vi "Write-OSP-J-t.vi"(8 "Init cluster":T1, 11 "Array":dbl[][](array[numeric])) -> ()   [LabVIEW 2020]
uses:
  <vilib>/Utility/file.llb/Write Delimited Spreadsheet (DBL).vi
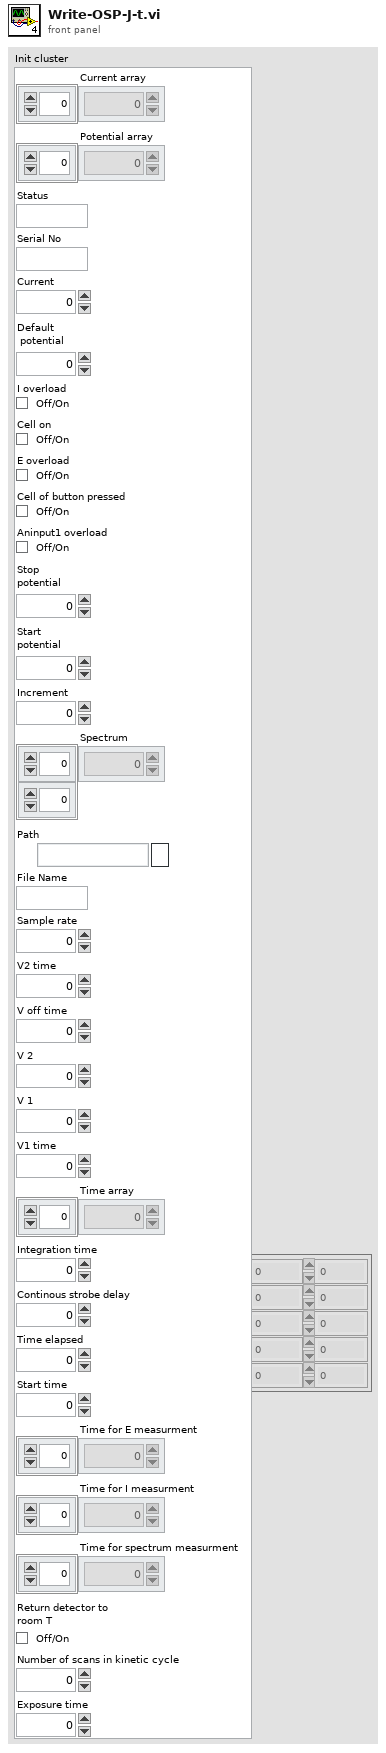
[diagram p1: front panel]
types:
  T1 = cluster{"Current array":dbl[], "Potential array":dbl[], "Status":string, "Serial No":string, "Current":dbl, "Default\n potential":dbl, "I overload":bool, "Cell on":bool, "E overload":bool, "Cell of button pressed":bool, "Aninput1 overload":bool, "Stop \npotential":dbl, "Start \npotential":dbl, "Increment":dbl, "Spectrum":dbl[][], "Path":path, "File Name":string, "Sample rate":dbl, "V2 time":dbl, "V off time":dbl, "V 2":dbl, "V 1":dbl, "V1 time":dbl, "Time array":dbl[], "Integration time":i32, "Continous strobe delay":i32, "Time elapsed ":i32, "Start time":i32, "Time for E measurment":i32[], "Time for I measurment ":i32[], "Time for spectrum measurment":i32[], "Return detector to \nroom T":bool, "Number of scans in kinetic cycle":i32, "Exposure time":i32}
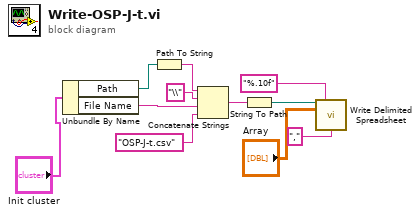
[diagram p0: block diagram]
diagram:
  n1 = Unbundle By Name("Init cluster") -> ("Path"=w11:path, "File Name"=w3:string)
  n2 = Path To String(path=w11) -> (string=w8:string)
  n3 = Concatenate Strings(w8, "\\" ("string"), w3, "OSP-J-t.csv") -> (w9:string)
  n4 = String To Path(string=w9) -> (path=w10:path)
  n5 = call-poly <vilib>:"Write Delimited Spreadsheet.vi"("file path (dialog if empty)"=w10, "format (%.3f)"="%.10f", "2D data"="Array", "delimiter (\\t)"="," ("delimiter (\\t)")) -> ()  [unwired: 10 in, 2 out]
